vi "MoveAbsSingleAxis.vi"(6 "Wait":bool=TRUE, 8 "error in (no error)":errorcluster, 9 "Value":dbl format="%.2f", 10 "Axis":i32=1, 11 "DLOwis in":refnum<class "DLOwis.lvclass">) -> (0 "error out":errorcluster, 3 "DLOwis out":refnum<class "DLOwis.lvclass">)   [LabVIEW 2019, in "DLOwis.lvclass"]
uses:
  DLOwis.lvclass
panel:
  out "Numeric":i32
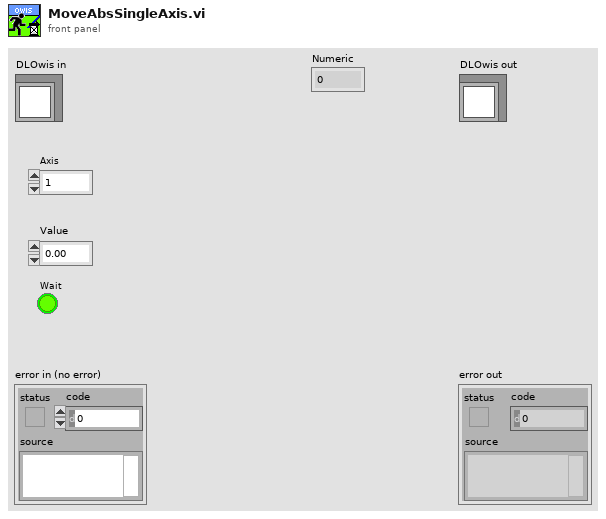
[diagram p1: front panel]
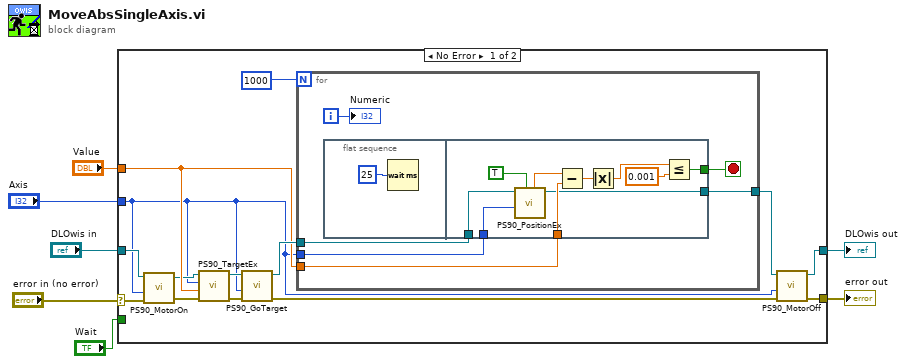
[diagram p0: block diagram]
diagram:
  n1 = case shown="No Error" "error in (no error)" {
    selector: "error in (no error)" -> [w13 w40]
    tunnel: [w9 w40] -> w6
    tunnel: "DLOwis in" -> [w16 w39]
    tunnel: "Axis" -> [w8 _]
    tunnel: [w11 w39] -> w4
    tunnel: "Wait" -> [_ _]
    tunnel: "Value" -> [w17 _]
    frame No Error {
      n2 = call "PS90_MotorOn.vi"("error in (no error)"=w13, "Axis number"=w8, "DLOwis.lvclass"=w16) -> ("error out"=w14:errorcluster, "DLOwis.lvclass"=w15:refnum<class "DLOwis.lvclass">)  [unwired: 2 in]
      n3 = call "PS90_TargetEx.vi"("error in (no error)"=w14, "dValue-In"=w17, "Axis number"=w8, "DLOwis.lvclass"=w15) -> ("error out"=w21:errorcluster, "DLOwis.lvclass"=w20:refnum<class "DLOwis.lvclass">)  [unwired: 5 in, 1 out]
      n4 = call "PS90_GoTarget.vi"("error in (no error)"=w21, "Axis number"=w8, "DLOwis.lvclass"=w20) -> ("error out"=w10:errorcluster, "DLOwis.lvclass"=w18:refnum<class "DLOwis.lvclass">)  [unwired: 7 in]
      n5 = for {
        N: 1000 -> [_]
        tunnel: w18 -> [w27]
        tunnel: w8 -> [w26]
        tunnel: w17 -> [w25]
        tunnel: [w22] -> w12
        i -> [w23]
        stop <- w24 stop-if-true
        n6 = flat-sequence {
          tunnel: w27 -> [w38]
          tunnel: w26 -> [w36]
          tunnel: w25 -> [w35]
          tunnel: [w30] -> w24
          tunnel: [w29] -> w22
          frame #0 {
            n7 = Wait (ms)(milliseconds to wait=u32 25) -> ()  [unwired: 1 out]
          }
          frame #1 {
            n8 = call "PS90_PositionEx.vi"("read?"=TRUE, "Axis number"=w36, "DLOwis.lvclass"=w38) -> ("DLOwis.lvclass"=w29:refnum<class "DLOwis.lvclass">, "dValue-Out"=w34:dbl)  [unwired: 5 in, 1 out]
            n9 = Subtract(x=w34, y=w35) -> (x-y=w33:dbl)
            n10 = Absolute Value(x=w33) -> (abs(x)=w32:dbl)
            n11 = Less Or Equal?(x=w32, y=0.001) -> (x <= y?=w30:bool)
          }
        }
        "Numeric" <- w23
      }
      n12 = call "PS90_MotorOff.vi"("error in (no error)"=w10, "Axis number"=w8, "DLOwis.lvclass"=w12) -> ("error out"=w9:errorcluster, "DLOwis.lvclass"=w11:refnum<class "DLOwis.lvclass">)  [unwired: 7 in]
    }
    frame Error {
    }
  }
  "error out" <- w6
  "DLOwis out" <- w4
